vi "CD Read Engine.vi"(5 "Inline Status Channels Refs":T1[](array[typedef]) format="%.0x", 7 "Error (in)":errorcluster, 8 "Output Channel Data []":T2[](array[typedef]) {"Labels Settings"."Label Timestamp Channel Data Reference" format="%.0x"; "Labels Settings"."Label Disable/Trigger Channel Reference" format="%.0x"; "Labels Settings"."Word"."Param Setting"."Item Refs" format="%.0x"; "Labels Settings"."Word"."Param Setting"."Num Bits" min=1 max=32; "Labels Settings"."Word"."Param Setting"."Start Bit" min=8 max=31; "Labels Settings"."Label" format="%.0o"}, 9 "Card Parameters (in)":T16) -> (0 "Error (out)":errorcluster)   [LabVIEW 2020, in "Ballard Arinc-429 Engine.lvlib"]
uses:
  Ballard Arinc-429 Engine.lvlib
  <instrlib>/BTICardLib/Public/Controls/429 Record.ctl
  <instrlib>/BTICardLib/Public/Controls/Seq Run Status.ctl
  <instrlib>/BTICardLib/Public/Controls/Seq Fill Status.ctl
  Shared/Controls and Global/RT HW Channel.ctl
  Shared/Controls and Global/RT Label Settings.ctl
  Shared/Controls and Global/Label.ctl
  Shared/Controls and Global/transferPeriod.ctl
  Shared/Controls and Global/RT Word Settings.ctl
  Shared/Controls and Global/RT Param Setting.ctl
  Shared/Controls and Global/Start Bit.ctl
  Shared/Controls and Global/Number of Bits.ctl
  <vilib>/NI VeriStand/Custom Device API/Block Data Reference.ctl
  <vilib>/NI VeriStand/Custom Device API/Data Reference.ctl
  <vilib>/NI VeriStand/Custom Device API/Custom Device Item Ref.ctl
  Shared/Controls and Global/TransferType.ctl
  RT Controls/Card Parameters.ctl
  Shared/Controls and Global/Initialization Method.ctl
  <instrlib>/BTICardLib/BTICardLV.lvlib
  <vilib>/NI VeriStand/Custom Device Tools/Custom Device Utility Library/Custom Device Utility Library.lvlib
  Shared/Ballard Arinc-429 Shared.lvlib
  <vilib>/NI VeriStand/Custom Device API/Custom Device API.lvlib
panel:
  in  "Tab Control":enum32{"Controls & Indicators", "Misc"}(tab)
  out "# of records read":i32
  out "Record []":T13[](array[typedef]) {"type" format="%04x"; "timestamp" format="%08x"; "msgact" format="%04x"; "data" format="%08x"; "timestamph" format="%08x"}
  out "run status":T14 items=["SEQ_STARTED", "SEQ_STOPPED", "SEQ_ERROR"]
  out "fill status":T15 items=["SEQ_EMPTY", "SEQ_PARTIAL", "SEQ_FULL"]
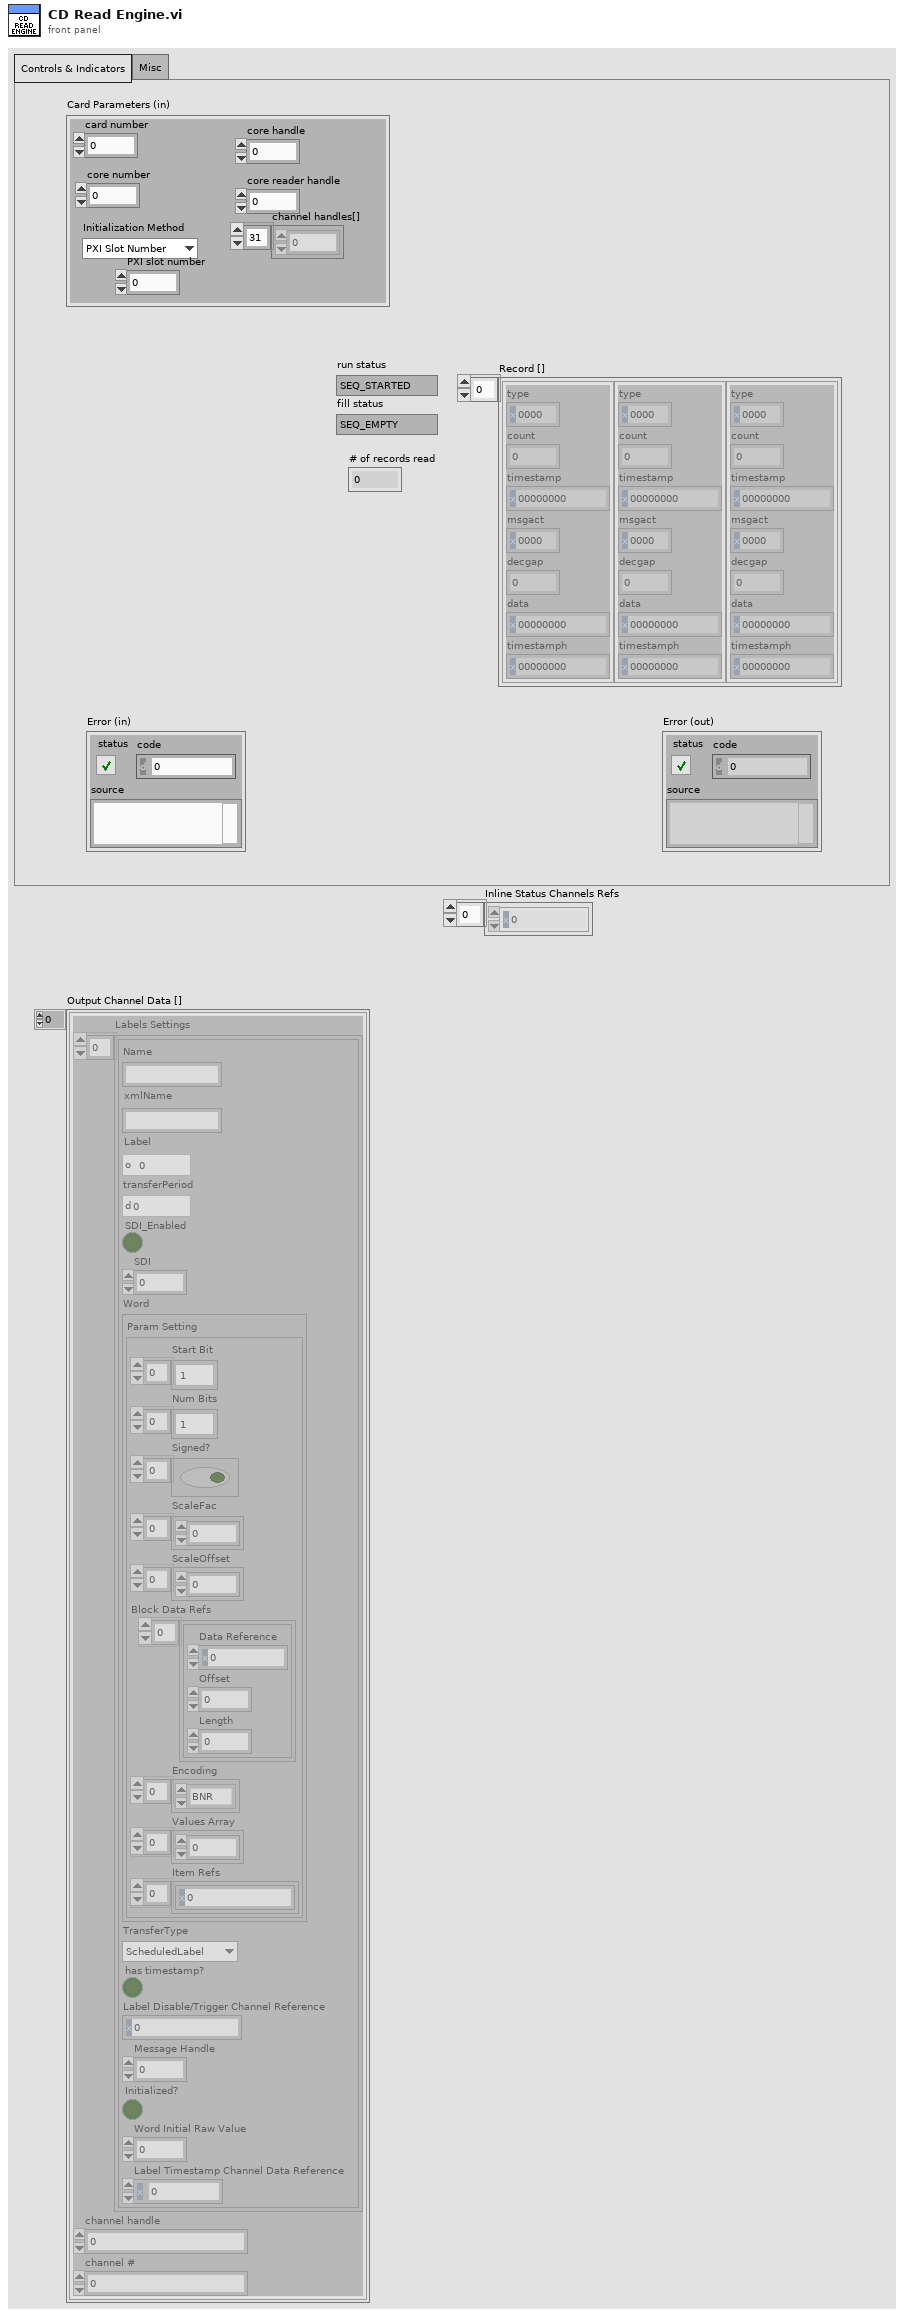
[diagram p1: front panel]
types:
  T1 = typedef "Custom Device API.lvlib/Data Reference.ctl" = i32
  T2 = typedef "Ballard Arinc-429 Shared.lvlib/RT HW Channel.ctl" = cluster{"Labels Settings":T3[], "channel handle":u64, "channel #":u16}
  T3 = typedef "Ballard Arinc-429 Shared.lvlib/RT Label Settings.ctl" = cluster{"Name":string, "xmlName":string, "Label":T4, "transferPeriod":T5, "SDI_Enabled":bool, "SDI":u8, "Word":T6, "TransferType":T12, "has timestamp?":bool, "Label Disable/Trigger Channel Reference":T11, "Message Handle":u64, "Initialized?":bool, "Word Initial Raw Value":u32, "Label Timestamp Channel Data Reference":T1}
  T4 = typedef "Ballard Arinc-429 Shared.lvlib/Label.ctl" = u8
  T5 = typedef "Ballard Arinc-429 Shared.lvlib/transferPeriod.ctl" = u32
  T6 = typedef "Ballard Arinc-429 Shared.lvlib/RT Word Settings.ctl" = cluster{"Param Setting":T7}
  T7 = typedef "Ballard Arinc-429 Shared.lvlib/RT Param Setting.ctl" = cluster{"Start Bit":T8[], "Num Bits":T9[], "Signed?":bool[], "ScaleFac":dbl[], "ScaleOffset":dbl[], "Block Data Refs":T10[], "Encoding":enum16{"BNR", "BCD", "Discrete"}[], "Values Array":dbl[], "Item Refs":T11[]}
  T8 = typedef "Ballard Arinc-429 Shared.lvlib/Start Bit.ctl" = i32
  T9 = typedef "Ballard Arinc-429 Shared.lvlib/Number of Bits.ctl" = i32
  T10 = typedef "Custom Device API.lvlib/Block Data Reference.ctl" = cluster{"Data Reference":T1, "Offset":u64, "Length":u64}
  T11 = typedef "Custom Device API.lvlib/Custom Device Item Ref.ctl" = u64
  T12 = typedef "Ballard Arinc-429 Shared.lvlib/TransferType.ctl" = enum16{"ScheduledLabel", "Acyclic", "Block", "Strobe"}
  T13 = typedef "BTICardLV.lvlib/429 Record.ctl" = cluster{"type":u16, "count":u16, "timestamp":u32, "msgact":u16, "decgap":u16, "data":u32, "timestamph":u32}
  T14 = typedef "BTICardLV.lvlib/Seq Run Status.ctl" = u32
  T15 = typedef "BTICardLV.lvlib/Seq Fill Status.ctl" = u32
  T16 = typedef "Ballard Arinc-429 Engine.lvlib/Card Parameters.ctl" = cluster{"card number":i32, "core number":i32, "core handle":u64, "core reader handle":u64, "channel handles[]":u64[], "Initialization Method":T17, "PXI slot number":i32}
  T17 = typedef "Ballard Arinc-429 Shared.lvlib/Initialization Method.ctl" = enum16{"PXI Slot Number", "Card Number"}
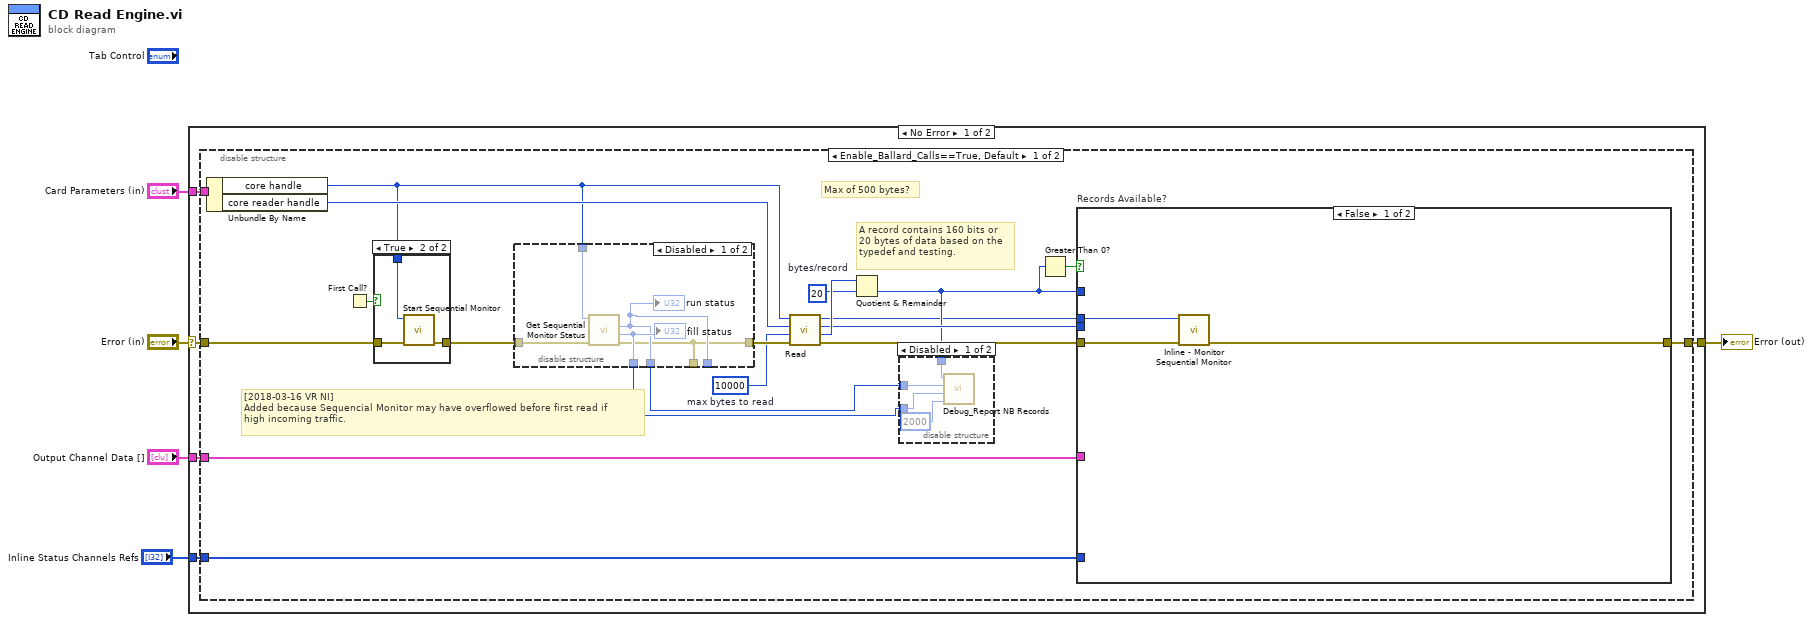
[diagram p0: block diagram]
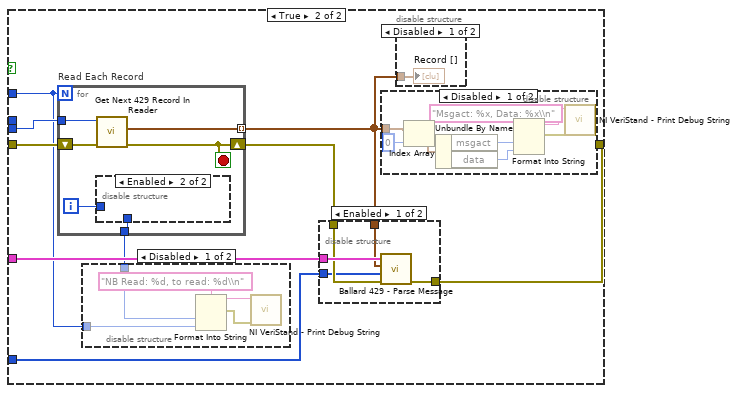
[diagram p5: hidden frame]
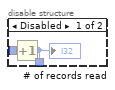
[diagram p10: hidden frame]
diagram:
  n1 = case shown="No Error" "Error (in)" {
    selector: "Error (in)" -> [w7 w86]
    tunnel: "Card Parameters (in)" -> [w10 _]
    tunnel: "Output Channel Data []" -> [w9 _]
    tunnel: [w8 w86] -> w3
    tunnel: "Inline Status Channels Refs" -> [w6 _]
    frame No Error {
      n2 = disable-structure shown="Enable_Ballard_Calls==True, Default" {
        disable-tunnel: w10 -> [w22 _]
        disable-tunnel: w9 -> [w21 _]
        disable-tunnel: [w20 w85] -> w8
        disable-tunnel: w7 -> [w17 w85]
        disable-tunnel: w6 -> [w12 _]
        frame condition #0 (active) {
          w26 = 20  # bytes/record
          w28 = 10000  # max bytes to read
          # "[2018-03-16 VR NI]\nAdded because Sequencial Monitor may have overflowed before first read if\nhigh incoming traffic."
          # "A record contains 160 bits or 20 bytes of data based on the typedef and testing."
          # "Max of 500 bytes?"
          n3 = Unbundle By Name(w22) -> ("core handle"=w13:u64, "core reader handle"=w30:u64)
          n4 = First Call?() -> (First Call?: T/F=w15:bool)
          n5 = case shown="True" w15 {
            tunnel: w13 -> [_ w34]
            tunnel: w17 -> [w31 w33]
            tunnel: [w31 w32] -> w16
            frame False {
            }
            frame True {
              n6 = call <instrlib>:"Start Sequential Monitor.vi"("error in (no error)"=w33, "core handle in"=w34) -> ("error out"=w32:errorcluster)  [unwired: 8 in, 1 out]
            }
          }
          n7 = disable-structure shown="Disabled" {
            disable-tunnel: w13 -> [w43 _]
            disable-tunnel: w16 -> [w42 w44]
            disable-tunnel: [w39 w44] -> w29
            disable-tunnel: [w40 _] -> w19
            disable-tunnel: [w41 _] -> w18
            disable-tunnel: [w40 _] -> _
            disable-tunnel: [w39 _] -> _
            frame Disabled {
              n8 = call <instrlib>:"Get Sequential Monitor Status.vi"("error in (no error)"=w42, "core handle in"=w43) -> ("error out"=w39:errorcluster, "fill status"=w41:T15, "run status"=w40:T14)  [unwired: 6 in, 1 out]
              "run status" <- w40
              "fill status" <- w41
            }
            frame Enabled {
            }
          }
          n9 = call <instrlib>:"Read.vi"("error in (no error)"=w29, "max bytes to read"=w28, "core reader handle in"=w30, "core handle in"=w13) -> ("error out"=w23:errorcluster, "bytes read"=w27:i32, "core reader handle out"=w24:u64, "core handle out"=w11:u64)  [unwired: 4 in]
          n10 = Quotient & Remainder(x=w27, y=w26) -> (floor(x/y)=w14:i32)  [unwired: 1 out]
          n11 = disable-structure shown="Disabled" {
            disable-tunnel: w14 -> [w38 _]
            disable-tunnel: w19 -> [w36 _]
            disable-tunnel: w18 -> [w35 _]
            frame Disabled {
              n12 = call "Debug_Report NB Records.vi"("Decimation"=2000, "fill status"=w35, "run status"=w36, "NB of Records Available"=w38) -> ()  [unwired: 8 in]
            }
            frame Enabled {
            }
          }
          n13 = Greater Than 0?(x=w14) -> (x > 0?=w25:bool)
          n14 = case "Records Available?" shown="False" w25 {
            tunnel: w23 -> [w47 w56]
            tunnel: [w46 w53] -> w20
            tunnel: w24 -> [_ w55]
            tunnel: w14 -> [_ w50]
            tunnel: w21 -> [_ w54]
            tunnel: w12 -> [_ w48]
            tunnel: w11 -> [w45 _]
            frame False {
              n15 = call "Inline - Monitor Sequential Monitor.vi"("error in (no error)"=w47, "core handle in"=w45) -> ("error out"=w46:errorcluster)  [unwired: 8 in, 1 out]
            }
            frame True {
              n16 = for "Read Each Record" {
                N: w50 -> [_]
                tunnel: w55 -> [w81]
                tunnel: [w79] -> w49 mode=indexing
                shift-right: [w78] -> w52
                shift-left: w56 -> [w82]
                tunnel: [w77] -> w51
                i -> [w80]
                stop <- w78 stop-if-true
                n17 = call <instrlib>:"Get Next 429 Record In Reader.vi"("error in (no error)"=w82, "core reader handle in"=w81) -> ("error out"=w78:errorcluster, "record out"=w79:T13)  [unwired: 7 in, 1 out]
                n18 = disable-structure shown="Enabled" {
                  disable-tunnel: w80 -> [w84 _]
                  disable-tunnel: [w83 _] -> w77
                  frame Disabled {
                    n19 = Increment(x=w84) -> (x+1=w83:i32)
                    "# of records read" <- w83
                  }
                  frame Enabled {
                  }
                }
              }
              n20 = disable-structure shown="Disabled" {
                disable-tunnel: w51 -> [w73 _]
                disable-tunnel: w50 -> [w72 _]
                frame Disabled {
                  n21 = Format Into String(format string="NB Read: %d, to read: %d\\n", w73, w72) -> (resulting string=w71:string, error out=w75:errorcluster)  [unwired: 2 in]
                  n22 = call <vilib>:"NI VeriStand - Print Debug String.vi"("error in (no error)"=w75, "Message"=w71) -> ()  [unwired: 9 in, 1 out]
                }
                frame Enabled {
                }
              }
              n23 = disable-structure shown="Enabled" {
                disable-tunnel: w54 -> [w61 _]
                disable-tunnel: [w60 w62] -> w53
                disable-tunnel: w52 -> [w59 w62]
                disable-tunnel: w49 -> [w58 _]
                disable-tunnel: w48 -> [w57 _]
                frame Enabled {
                  n24 = call "Ballard 429 - Parse Message.vi"("Error (in)"=w59, "Inline Status Channels Refs"=w57, "Record []"=w58, "Channel Data [] In"=w61) -> ("Error (out)"=w60:errorcluster)  [unwired: 7 in]
                }
                frame Disabled {
                }
              }
              n25 = disable-structure shown="Disabled" {
                disable-tunnel: w49 -> [w70 _]
                frame Disabled {
                  n26 = Index Array(array=w70, index=0) -> (element=w68:T13)
                  n27 = Unbundle By Name(w68) -> ("msgact"=w67:u16, "data"=w66:u32)
                  n28 = Format Into String(format string="Msgact: %x, Data: %x\\n", w67, w66) -> (resulting string=w64:string, error out=w65:errorcluster)  [unwired: 2 in]
                  n29 = call <vilib>:"NI VeriStand - Print Debug String.vi"("error in (no error)"=w65, "Message"=w64) -> ()  [unwired: 9 in, 1 out]
                }
                frame Enabled {
                }
              }
              n30 = disable-structure shown="Disabled" {
                disable-tunnel: w49 -> [w76 _]
                frame Disabled {
                  "Record []" <- w76
                }
                frame Enabled {
                }
              }
            }
          }
        }
        frame condition #1 {
        }
      }
    }
    frame Error {
    }
  }
  "Error (out)" <- w3
